vi "Test_WriteItemName_NoValue_ListAll_NameReturned.vi"(8 "error in (no error)":errorcluster, 11 "TestCase in":refnum<class "TestComposedLookupTable.lvclass">) -> (0 "error out":errorcluster, 3 "TestCase out":refnum<class "TestComposedLookupTable.lvclass">)   [LabVIEW 2017, in "TestComposedLookupTable.lvclass"]
uses:
  TestComposedLookupTable.lvclass
  Source/LookupTable/LookupTable.lvclass/LookupTable.ctl
  87404576-7c1b-47e7-8bc2-e5fc3b6d3934.vi
  Source/LookupTable/Read Table Reference.vi
  87404576-7c1b-47e7-8bc2-e5fc3b6d3934.vi/01d66347-55e8-4add-badd-9a774484aa6f.vi
  Source/LookupTable/LookupTable.lvclass
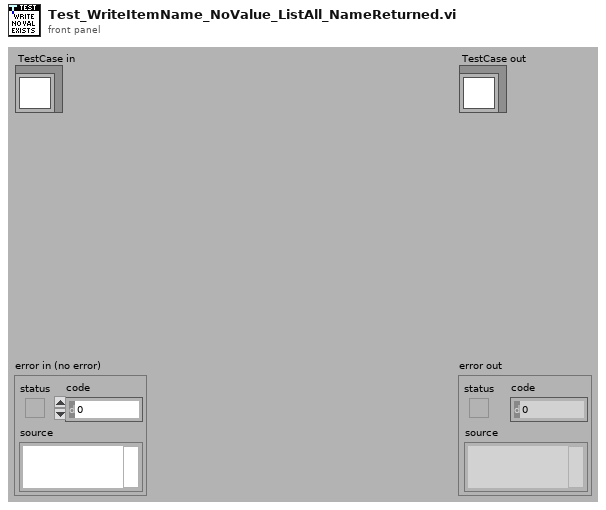
[diagram p1: front panel]
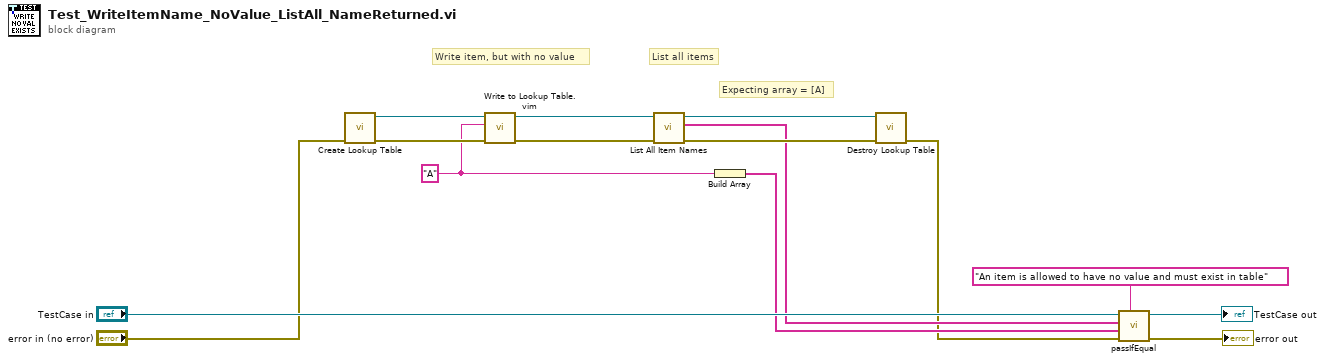
[diagram p0: block diagram]
diagram:
  w4 = "A" ("Item Name")
  # "Expecting array = [A]"
  # "List all items"
  # "Write item, but with no value"
  n1 = call "Create Lookup Table.vi"("error in (no error)"="error in (no error)") -> ("error out"=w15:errorcluster, "LookupTable Reference"=w8:refnum<data-value>)  [unwired: 9 in]
  n2 = call "Write to Lookup Table.vim"("error in (no error)"=w15, "Item Name"=w4, "LookupTable Reference"=w8) -> ("error out"=w9:errorcluster, "LookupTable Reference Out"=w6:refnum<data-value>)  [unwired: 6 in, 1 out]
  n3 = call "List All Item Names.vi"("error in (no error)"=w9, "LookupTable Reference"=w6) -> ("error out"=w7:errorcluster, "All Items"=w5:string[], "LookupTable Reference Out"=w10:refnum<data-value>)  [unwired: 6 in, 1 out]
  n4 = Build Array(w4) -> (w3:string[])
  n5 = call "Destroy Lookup Table.vi"("error in (no error)"=w7, "LookupTable Reference"=w10) -> ("error out"=w2:errorcluster)  [unwired: 9 in]
  n6 = call-dynamic "passIfEqual.vi"("custom report message (\"\")"="An item is allowed to have no value and must exist in table" ("custom report message (\"\")"), "error in (no error)"=w2, "y"=w3, "x"=w5, "TestCase in"="TestCase in") -> ("error out"=→"error out":errorcluster, "TestCase out"=→"TestCase out":refnum<class "TestComposedLookupTable.lvclass">)  [unwired: 5 in]
